vi "ColorDecoder.vi"() -> ()   [LabVIEW 2018]
panel:
  in  "Color":u32(colorbox)
  out "Resolved Color":u32
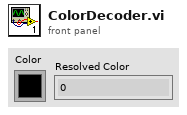
[diagram p1: front panel]
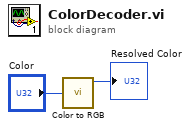
[diagram p0: block diagram]
diagram:
  n1 = call <vilib>:"Color to RGB.vi"("Color"="Color") -> ("Resolved Color"=→"Resolved Color":u32)  [unwired: 3 out]
